vi "Draw Textured Triangle v2.vi"(0 "Texture 3":T1, 4 "Texture 2":T1, 6 "Texture 1":T1, 7 "Texture":T2, 8 "Point 3":T1={"x"=60, "y"=100}, 9 "Point 2":T1={"x"=80, "y"=80}, 10 "Point 1":T1={"x"=20, "y"=20}) -> (3 "Pixel Data out":u32[][](array[numeric]))   [LabVIEW 2022 SP3, in "Raster.lvlib"]
uses:
  Raster.lvlib
  Point 2D.ctl
  <vilib>/picture/picture.llb/imagedata.ctl
  Screen Dimensions.ctl
  <vilib>/Utility/miscctls.llb/LVPointTypeDef.ctl
  Utility/Convert Pixels To Picture.vi/d601d993-a776-4dc8-89c7-357d8398c88c.vi
  Utility/Convert Pixels To Picture.vi/7816d0d6-8e4d-41a2-85ac-ed82f1435763.vi
  <vilib>/Utility/High Resolution Relative Seconds.vi
  <vilib>/picture/picture.llb/Draw Unflattened Pixmap.vi
  <vilib>/picture/picture.llb/Draw True-Color Pixmap.vi
  Utility/Utility.lvlib
panel:
  out "Array":u32[](array[colorbox])
  in  "Path":path
  out "Point 4":T1
  out "2D Picture 2":picture
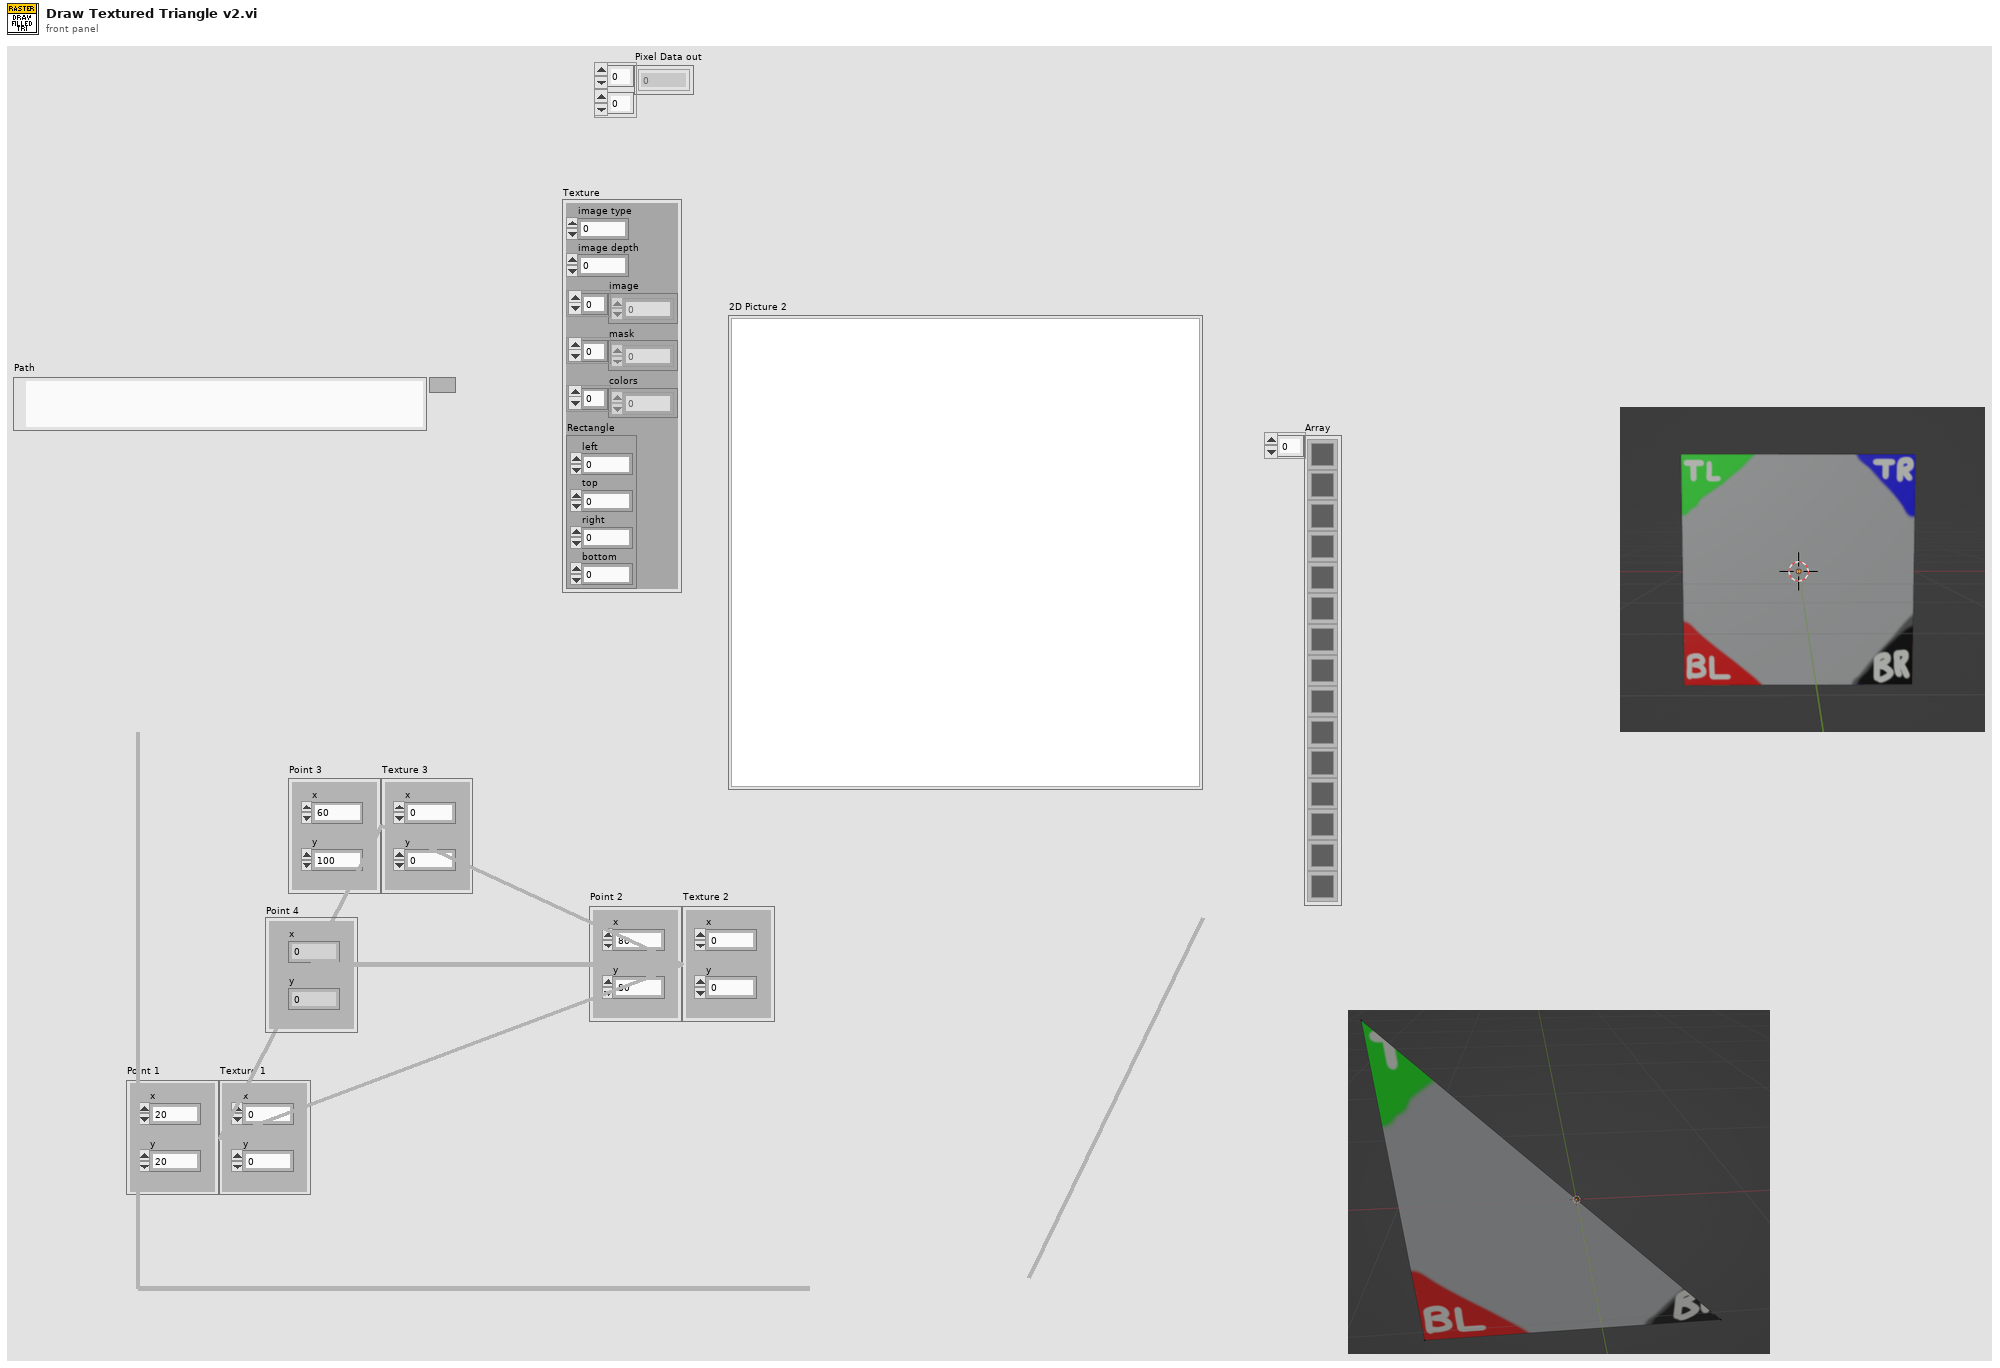
[diagram p1: front panel]
types:
  T1 = typedef "Raster.lvlib/Point 2D.ctl" = cluster{"x":i32, "y":i32}
  T2 = typedef "imagedata.ctl" = cluster{"image type":i32, "image depth":i32, "image":u8[], "mask":u8[], "colors":u32[], "Rectangle":cluster{"left":i16, "top":i16, "right":i16, "bottom":i16}}
  T3 = typedef "LVPointTypeDef.ctl" = cluster{"Horizontal":i16, "Vertical":i16}
  T4 = typedef "Raster.lvlib/Screen Dimensions.ctl" = cluster{"Width":u32, "Height":u32}
  T5 = cluster{"Texture 1":T1, "Texture 2":T1, "Texture 3":T1}
  T6 = typedef "Raster.lvlib/Line Parameters.ctl" = cluster{"1/m":dbl, "c":dbl}
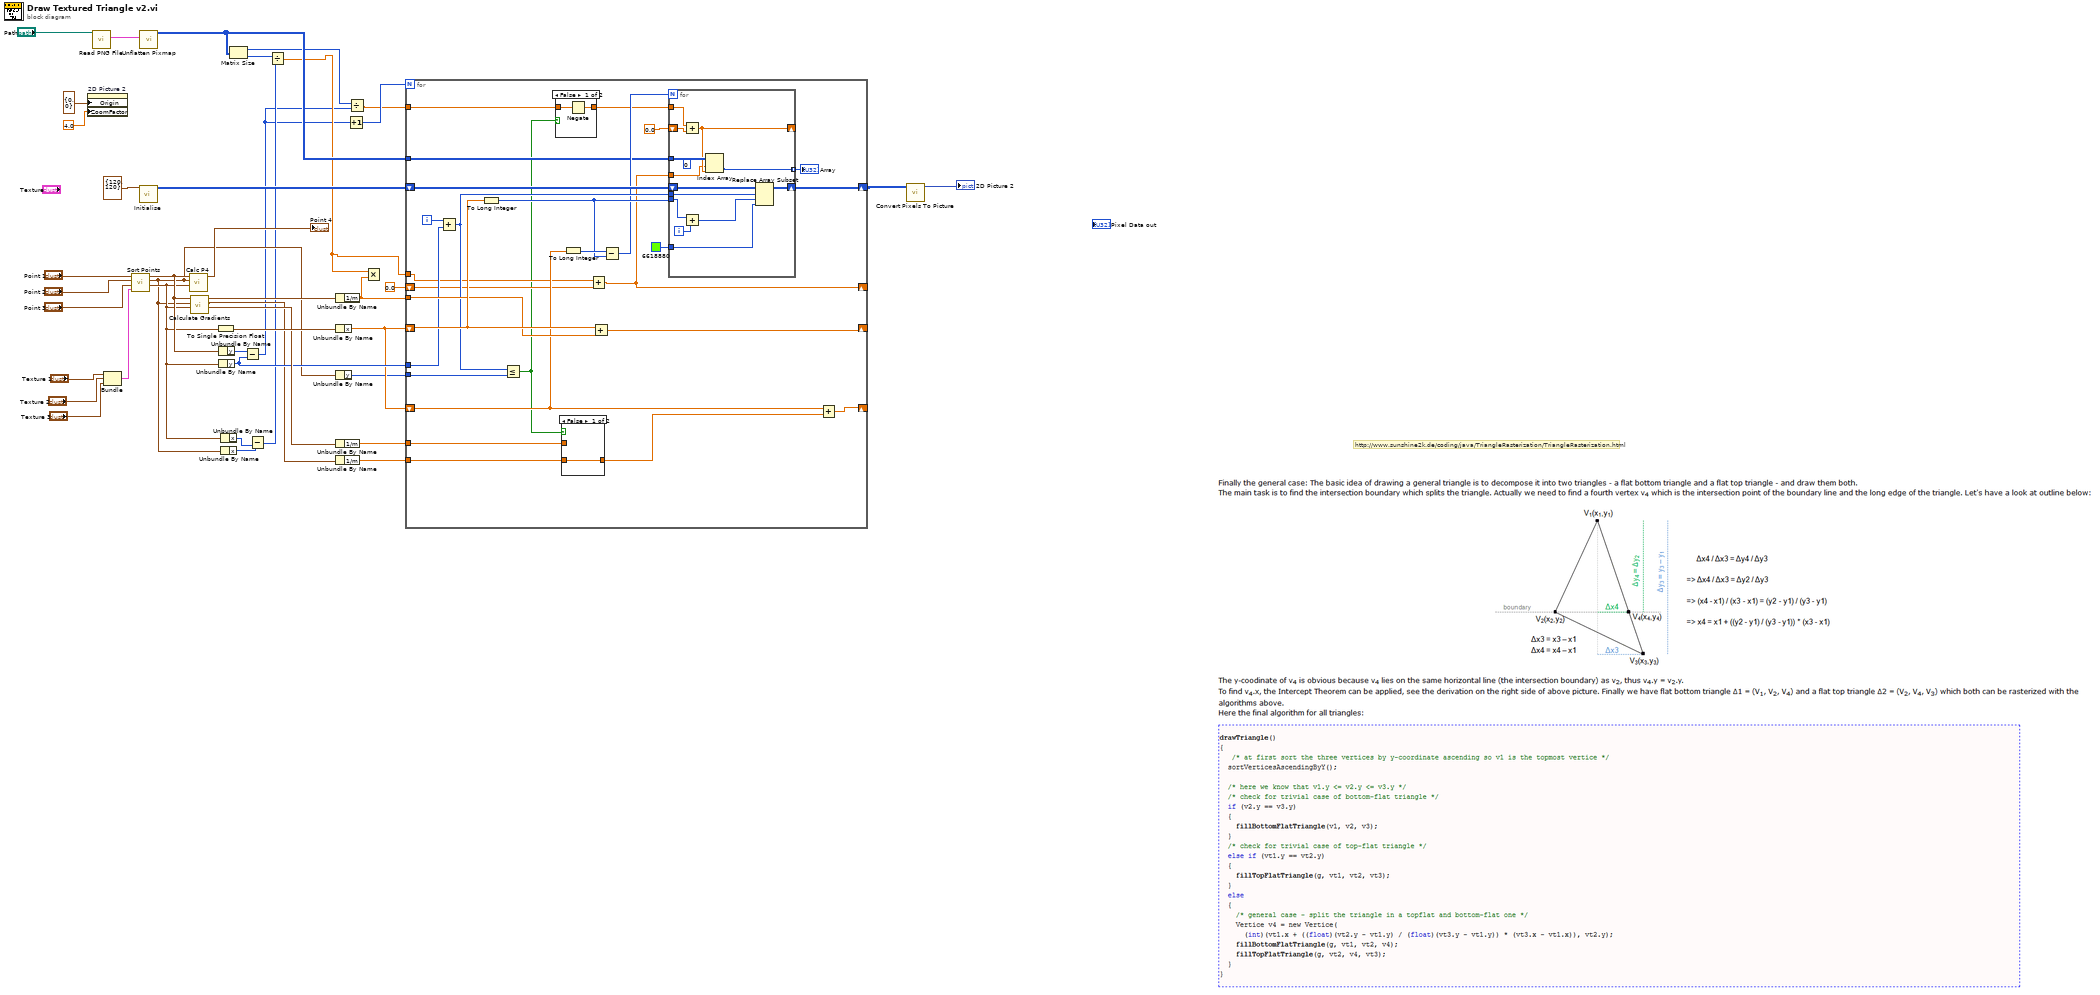
[diagram p0: block diagram]
diagram:
  # "http://www.sunshine2k.de/coding/java/TriangleRasterization/TriangleRasterization.html"
  n1 = property on="2D Picture 2" class="Pict"("Origin"=T3 {"Horizontal"=0, "Vertical"=0}, "ZoomFactor"=sgl 4.0 ("Zoom Factor")) -> ()  [unwired: 2 in, 2 out]
  n2 = call <vilib>:"Read PNG File.vi"("path to PNG file"="Path") -> ("image data"=w15:T2)  [unwired: 8 in, 2 out]
  n3 = Bundle("Texture 1"="Texture 1", "Texture 2"="Texture 2", "Texture 3"="Texture 3") -> (w34:T5)  [unwired: 1 in]
  n4 = call "Sort Points.vi"("Texture Vertices"=w34, "Point 3"="Point 3", "Point 2"="Point 2", "Point 1"="Point 1") -> ("Bottom"=w14:T1, "Middle"=w13:T1, "Top"=w29:T1)  [unwired: 4 in, 1 out]
  n5 = call "Initialise.vi"("Screen Dimensions"=T4 {"Width"=120, "Height"=120}) -> ("Pixel Data out"=w31:u32[][])  [unwired: 10 in]
  n6 = call <vilib>:"Unflatten Pixmap.vi"("image data"=w15) -> ("24-bit pixmap"=w10:u32[][])  [unwired: 4 in, 6 out]
  n7 = call "Calc P4.vi"("Bottom"=w14, "Middle"=w13, "Top"=w29) -> ("Point 4"=→"Point 4":T1)  [unwired: 8 in]
  n8 = call "Calculate Gradients.vi"("Bottom"=w14, "Middle"=w13, "Top"=w29) -> ("Middle --> Bottom"=w26:T6, "Line Top --> Middle"=w20:T6, "Line Top --> Bottom"=w27:T6)  [unwired: 6 in]
  n9 = To Single Precision Float(number=w14) -> (single precision float=w28:cluster{"x":sgl, "y":sgl})
  n10 = Unbundle By Name(w29) -> ("y"=w33:i32)
  n11 = Unbundle By Name(w14) -> ("y"=w23:i32)
  n12 = Unbundle By Name(w14) -> ("x"=w12:i32)
  n13 = Unbundle By Name(w13) -> ("x"=w11:i32)
  n14 = Matrix Size(0:w10) -> (1:w3:i32, 2:w9:i32)
  n15 = Subtract(x=w33, y=w23) -> (x-y=w2:i32)
  n16 = Subtract(x=w11, y=w12) -> (x-y=w8:i32)
  n17 = Divide(x=w9, y=w8) -> (x/y=w4:dbl)
  n18 = Unbundle By Name(w27) -> ("1/m"=w7:dbl)
  n19 = Unbundle By Name(w28) -> ("x"=w21:sgl)
  n20 = Unbundle By Name(w13) -> ("y"=w17:i32)
  n21 = Unbundle By Name(w26) -> ("1/m"=w22:dbl)
  n22 = Unbundle By Name(w20) -> ("1/m"=w19:dbl)
  n23 = Increment(x=w2) -> (x+1=w5:i32)
  n24 = Divide(x=w3, y=w2) -> (x/y=w1:dbl)
  n25 = Multiply(x=w4, y=w7) -> ()  [unwired: 1 out]
  n26 = for {
    N: w5 -> [_]
    shift-right: [w62] -> w30
    shift-left: w31 -> [w68]
    shift-right: [w66] -> _
    shift-left: w21 -> [w67]
    tunnel: w7 -> [w65]
    tunnel: w23 -> [w63]
    shift-right: [w58] -> _
    shift-left: w21 -> [w52]
    tunnel: w22 -> [w61]
    tunnel: w19 -> [w57]
    tunnel: w17 -> [w59]
    tunnel: w10 -> [w48]
    tunnel: w4 -> [w49]
    shift-right: [w47] -> _
    shift-left: 0.0 ("1/m") -> [w50]
    tunnel: w1 -> [w43]
    i -> [w64]
    n27 = Add(x=w64, y=w63) -> (x+y=w60:i32)
    n28 = To Long Integer(number=w67) -> (32bit integer=w54:i32)
    n29 = Less Or Equal?(x=w60, y=w59) -> (x <= y?=w44:bool)
    n30 = case shown="False" w44 {
      tunnel: w43 -> [w70 w71]
      tunnel: [w69 w71] -> w42
      frame False {
        n31 = Negate(x=w70) -> (-x=w69:dbl)
      }
      frame True {
      }
    }
    n32 = case shown="False" w44 {
      tunnel: w61 -> [_ w86]
      tunnel: w57 -> [w85 _]
      tunnel: [w85 w86] -> w56
      frame False {
      }
      frame True {
      }
    }
    n33 = To Long Integer(number=w52) -> (32bit integer=w55:i32)
    n34 = Add(x=w49, y=w50) -> (x+y=w47:dbl)
    n35 = Add(x=w67, y=w65) -> (x+y=w66:dbl)
    n36 = Subtract(x=w55, y=w54) -> (x-y=w51:i32)
    n37 = for {
      N: w51 -> [_]
      tunnel: w60 -> [w82]
      tunnel: w54 -> [w81]
      shift-right: [w83] -> w62
      shift-left: w68 -> [w84]
      tunnel: u32 6618880 ("new element/subarray") -> [w72]
      tunnel: w48 -> [w78]
      tunnel: w47 -> [w73]
      tunnel: [w77] -> w46 mode=indexing
      tunnel: w42 -> [w76]
      shift-right: [w74] -> _
      shift-left: 0.0 ("1/m") -> [w75]
      i -> [w80]
      (unwired) 0 ("disabled index (row)")
      n38 = Add(x=w76, y=w75) -> (x+y=w74:dbl)
      n39 = Add(x=w81, y=w80) -> (x+y=w79:i32)
      n40 = Index Array(array=w78, index (row)=w73, index (col)=w74) -> (element=w77:u32)
      n41 = Replace Array Subset(array=w84, new element=w72, index (row)=w82, index (col)=w79) -> (w83:u32[][])
    }
    "Array" <- w46
    n42 = Add(x=w52, y=w56) -> (x+y=w58:dbl)
  }
  n43 = call "Convert Pixels To Picture.vi"("Pixel Data in"=w30) -> ("2D Picture"=→"2D Picture 2":picture)  [unwired: 9 in, 1 out]
